vi "Update Incoming Section.vi"(8 "error in (no error)":errorcluster, 10 "Outgoing":T2 {"Frames to Update"."Node Ref" format="%.0x"; "Frames to Delete" format="%.0x"}, 11 "Item Ref in":T1 format="%.0x") -> (0 "error out":errorcluster, 3 "Item Ref out":T1 format="%.0x")   [LabVIEW 2025, in "Protection and Counter Addon System Explorer.lvlib"]
uses:
  Protection and Counter Addon System Explorer.lvlib
  Types/VS Update List.ctl
  <vilib>/NI VeriStand/Custom Device API/Custom Device Item Ref.ctl
  Types/Base Frame Info_NoVS.ctl
  Types/Signal Attributes.ctl
  Types/CAN Filter Type.ctl
  Types/CAN Frame Update Results.ctl
  <vilib>/NI VeriStand/Custom Device Tools/Custom Device Utility Library/Search Direction.ctl
  <vilib>/NI VeriStand/Custom Device API/Custom Device Channel.ctl
  <vilib>/NI VeriStand/Custom Device API/Custom Device Channel Type.ctl
  Addon Shared/SubVIs/GUID Lookup.vi
  <vilib>/NI VeriStand/Custom Device Tools/Custom Device Utility Library/NI VeriStand - Search for Item by GUID.vi
  <vilib>/NI/NI VeriStand Advanced SysDef API/_SubVIs/SysDef.Property.Set.U32.vi
  <vilib>/NI/NI VeriStand Advanced SysDef API/_SubVIs/SysDef.Search.Name.vi
  <vilib>/NI/NI VeriStand Advanced SysDef API/SysDef API/Advanced System Definition.lvlib
  Addon Shared/Protection and Counter Addon Shared.lvlib
  <vilib>/NI VeriStand/Custom Device API/Custom Device API.lvlib
  <vilib>/NI VeriStand/Custom Device Tools/Custom Device Utility Library/Custom Device Utility Library.lvlib
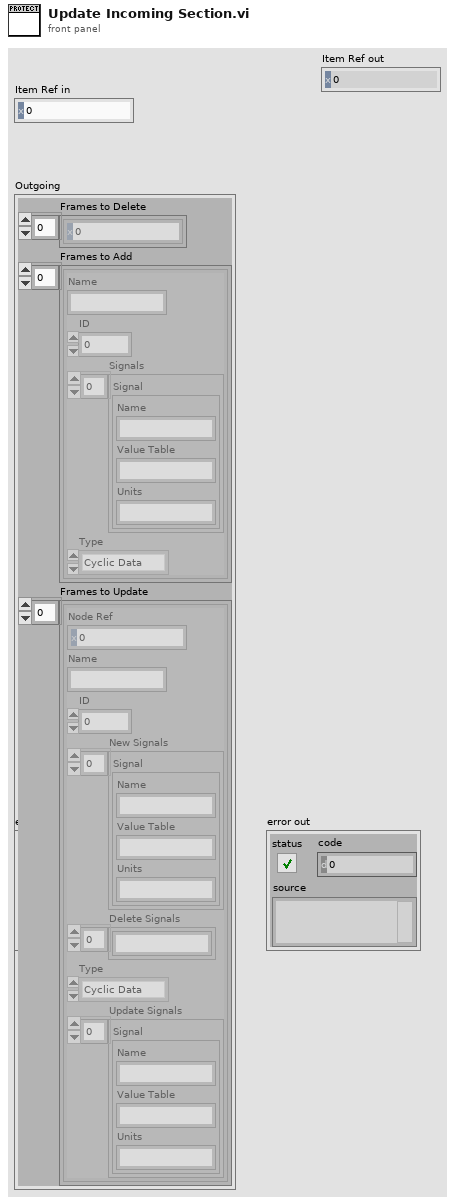
[diagram p1: front panel]
types:
  T1 = typedef "Custom Device API.lvlib/Custom Device Item Ref.ctl" = u64
  T2 = typedef "Protection and Counter Addon System Explorer.lvlib/VS Update List.ctl" = cluster{"Frames to Delete":T1[], "Frames to Add":T3[], "Frames to Update":T6[]}
  T3 = typedef "Protection and Counter Addon System Explorer.lvlib/Base Frame Info_NoVS.ctl" = cluster{"Name":string, "ID":u32, "Signals":T4[], "Type":T5}
  T4 = typedef "Protection and Counter Addon System Explorer.lvlib/Signal Attributes.ctl" = cluster{"Name":string, "Value Table":string, "Units":string}
  T5 = typedef "Protection and Counter Addon System Explorer.lvlib/CAN Filter Type.ctl" = enum16{"Cyclic Data", "Event Data", "Cyclic/Event", "All"}
  T6 = typedef "Protection and Counter Addon System Explorer.lvlib/CAN Frame Update Results.ctl" = cluster{"Node Ref":T1, "Name":string, "ID":u32, "New Signals":T4[], "Delete Signals":string[], "Type":T5, "Update Signals":T4[]}
  T7 = typedef "Custom Device Utility Library.lvlib/Search Direction.ctl" = enum16{"Down", "Up"}
  T8 = typedef "Custom Device API.lvlib/Custom Device Channel.ctl" = cluster{"Type":T9, "Units":string, "Default Value":dbl, "Faultable":bool, "Scalable":bool}
  T9 = typedef "Custom Device API.lvlib/Custom Device Channel Type.ctl" = enum16{"Input", "Output"}
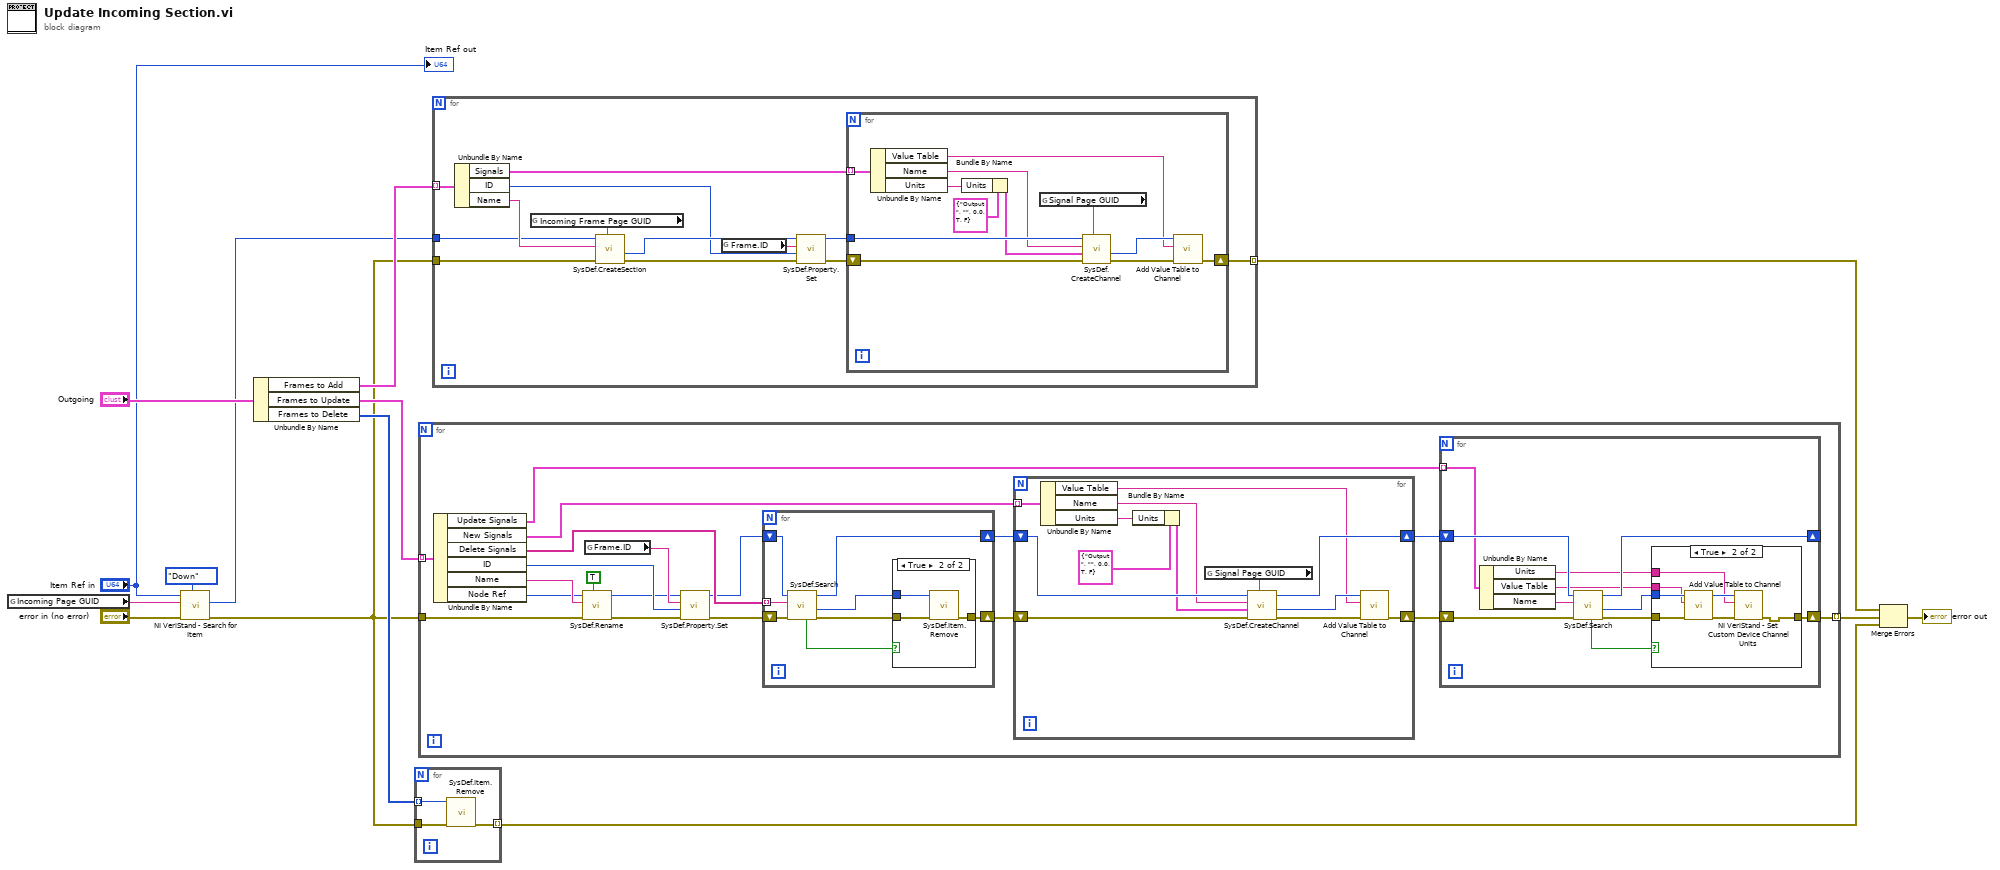
[diagram p0: block diagram]
diagram:
  n1 = global read "GUID Lookup.vi" "Incoming Page GUID"() -> (w3:string)
  n2 = call-poly <vilib>:"NI VeriStand - Search for Item.vi"("Direction (Down)"=Search_Direction."Down", "error in"="error in (no error)", "Item GUID"=w3, "Section Ref in"="Item Ref in") -> ("error out"=w1:errorcluster, "Item Ref"=w2:T1)  [unwired: 4 in, 2 out]
  n3 = Unbundle By Name("Outgoing") -> ("Frames to Add"=w13:T3[], "Frames to Update"=w12:T6[], "Frames to Delete"=w11:T1[])
  n4 = for {
    tunnel: w11 -> [w15] mode=indexing
    tunnel: w1 -> [w17]
    tunnel: [w16] -> w8 mode=indexing
    n5 = call <vilib>:"SysDef.Item.Remove.vi"("error in (no error)"=w17, "nodeID"=w15) -> ("error out"=w16:errorcluster)  [unwired: 8 in, 1 out]
  }
  n6 = for {
    tunnel: w12 -> [w36] mode=indexing
    tunnel: w1 -> [w22]
    tunnel: [w20] -> w7 mode=indexing
    n7 = Unbundle By Name(w36) -> ("Update Signals"=w18:T4[], "New Signals"=w31:T4[], "Delete Signals"=w32:string[], "ID"=w34:u32, "Name"=w35:string, "Node Ref"=w23:T1)
    n8 = call <vilib>:"SysDef.Rename.vi"("Force Rename (F)"=TRUE, "error in (no error)"=w22, "Name"=w35, "nodeID"=w23) -> ("error out"=w29:errorcluster, "nodeID out"=w30:u64)  [unwired: 5 in, 1 out]
    n9 = global read "GUID Lookup.vi" "Frame.ID"() -> (w33:string)
    n10 = call-poly <vilib>:"SysDef.Property.Set.vi"("error in (no error)"=w29, "Value"=w34, "Property Name"=w33, "nodeID"=w30) -> ("error out"=w25:errorcluster, "nodeID out"=w28:u64)  [unwired: 6 in]
    n11 = for {
      tunnel: w32 -> [w69] mode=indexing
      shift-right: [w72] -> w27
      shift-left: w28 -> [w76]
      shift-right: [w71] -> w26
      shift-left: w25 -> [w70]
      n12 = call-poly <vilib>:"SysDef.Search.vi"("error in (no error)"=w70, "Name"=w69, "nodeID"=w76) -> ("error out"=w73:errorcluster, "Value out"=w74:u64, "nodeID out"=w72:u64, "Found?"=w75:bool)  [unwired: 5 in]
      n13 = case shown="True" w75 {
        tunnel: w74 -> [_ w80]
        tunnel: w73 -> [w77 w79]
        tunnel: [w77 w78] -> w71
        frame False {
        }
        frame True {
          n14 = call <vilib>:"SysDef.Item.Remove.vi"("error in (no error)"=w79, "nodeID"=w80) -> ("error out"=w78:errorcluster)  [unwired: 8 in, 1 out]
        }
      }
    }
    n15 = for {
      shift-right: [w61] -> w21
      shift-left: w26 -> [w67]
      tunnel: w31 -> [w65] mode=indexing
      shift-right: [w64] -> w19
      shift-left: w27 -> [w68]
      n16 = Unbundle By Name(w65) -> ("Value Table"=w59:string, "Name"=w60:string, "Units"=w58:string)
      n17 = Bundle By Name(cluster=T8 {"Type"=enum."Output", "Units"="", "Default Value"=0.0, "Faultable"=TRUE, "Scalable"=FALSE} ("Channel"), "Units"=w58) -> (w56:T8)
      n18 = global read "GUID Lookup.vi" "Signal Page GUID"() -> (w66:string)
      n19 = call <vilib>:"SysDef.CreateChannel.vi"("GUID"=w66, "error in (no error)"=w67, "Channel"=w56, "Name"=w60, "nodeID"=w68) -> ("error out"=w62:errorcluster, "New NodeID"=w63:u64, "nodeID out"=w64:u64)  [unwired: 3 in, 1 out]
      n20 = call "Add Value Table to Channel.vi"("error in (no error)"=w62, "Value Table"=w59, "Channel Ref"=w63) -> ("error out"=w61:errorcluster)  [unwired: 7 in, 1 out]
    }
    n21 = for {
      tunnel: w18 -> [w40] mode=indexing
      shift-right: [w43] -> _
      shift-left: w19 -> [w47]
      shift-right: [w42] -> w20
      shift-left: w21 -> [w41]
      n22 = Unbundle By Name(w40) -> ("Units"=w37:string, "Value Table"=w38:string, "Name"=w39:string)
      n23 = call-poly <vilib>:"SysDef.Search.vi"("error in (no error)"=w41, "Name"=w39, "nodeID"=w47) -> ("error out"=w44:errorcluster, "Value out"=w45:u64, "nodeID out"=w43:u64, "Found?"=w46:bool)  [unwired: 5 in]
      n24 = case shown="True" w46 {
        tunnel: w45 -> [_ w54]
        tunnel: w44 -> [w48 w55]
        tunnel: [w48 w50] -> w42
        tunnel: w38 -> [_ w53]
        tunnel: w37 -> [_ w49]
        frame False {
        }
        frame True {
          n25 = call "Add Value Table to Channel.vi"("error in (no error)"=w55, "Value Table"=w53, "Channel Ref"=w54) -> ("error out"=w51:errorcluster, "Channel Ref out"=w52:u64)  [unwired: 7 in]
          n26 = call <vilib>:"NI VeriStand - Set Custom Device Channel Units.vi"("error in (no error)"=w51, "Units"=w49, "Channel Ref in"=w52) -> ("error out"=w50:errorcluster)  [unwired: 7 in, 1 out]
        }
      }
    }
  }
  n27 = for {
    tunnel: w13 -> [w93] mode=indexing
    tunnel: w1 -> [w83]
    tunnel: [w82] -> w6 mode=indexing
    tunnel: w2 -> [w81]
    n28 = Unbundle By Name(w93) -> ("Signals"=w86:T4[], "ID"=w91:u32, "Name"=w89:string)
    n29 = global read "GUID Lookup.vi" "Incoming Frame Page GUID"() -> (w84:string)
    n30 = call <vilib>:"SysDef.CreateSection.vi"("GUID"=w84, "error in (no error)"=w83, "Name"=w89, "nodeID"=w81) -> ("error out"=w90:errorcluster, "New NodeID"=w92:u64)  [unwired: 4 in, 2 out]
    n31 = global read "GUID Lookup.vi" "Frame.ID"() -> (w85:string)
    n32 = call-poly <vilib>:"SysDef.Property.Set.vi"("error in (no error)"=w90, "Value"=w91, "Property Name"=w85, "nodeID"=w92) -> ("error out"=w87:errorcluster, "nodeID out"=w88:u64)  [unwired: 6 in]
    n33 = for {
      tunnel: w88 -> [w105]
      tunnel: w86 -> [w103] mode=indexing
      shift-right: [w98] -> w82
      shift-left: w87 -> [w104]
      n34 = Unbundle By Name(w103) -> ("Value Table"=w97:string, "Name"=w101:string, "Units"=w96:string)
      n35 = Bundle By Name(cluster=T8 {"Type"=enum."Output", "Units"="", "Default Value"=0.0, "Faultable"=TRUE, "Scalable"=FALSE} ("Channel"), "Units"=w96) -> (w94:T8)
      n36 = global read "GUID Lookup.vi" "Signal Page GUID"() -> (w102:string)
      n37 = call <vilib>:"SysDef.CreateChannel.vi"("GUID"=w102, "error in (no error)"=w104, "Channel"=w94, "Name"=w101, "nodeID"=w105) -> ("error out"=w99:errorcluster, "New NodeID"=w100:u64)  [unwired: 3 in, 2 out]
      n38 = call "Add Value Table to Channel.vi"("error in (no error)"=w99, "Value Table"=w97, "Channel Ref"=w100) -> ("error out"=w98:errorcluster)  [unwired: 7 in, 1 out]
    }
  }
  n39 = Merge Errors(w6, w7, w8) -> (→"error out":errorcluster)
  "Item Ref out" <- "Item Ref in"
